vi "Begin.vi"(8 "error in":errorcluster) -> (0 "error out":errorcluster)   [LabVIEW 2016]
doc: "Called before other user functions, this VI is expected to open initial I/O refnums, load in file data, and do all program initialization. Notice that the <B>error out</B> terminal is simply used for data flow. Wiring it to other structures or subVIs ensures that this VI runs first."
uses:
  <vilib>/Rock Robotics/SystemInterfaces/i2clib/i2c_bus.ctl
  <vilib>/Rock Robotics/WPI/DriverStation/WPI_DriverStationRobotMode2.ctl
  <vilib>/Rock Robotics/WPI/Joystick/WPI_JoystickDeviceEnum.ctl
  <vilib>/Rock Robotics/SystemInterfaces/DIO/FPGA_DIOPWMChannel.ctl
  <vilib>/Rock Robotics/WPI/Solenoid/WPI_SolenoidChannel.ctl
  <vilib>/Rock Robotics/WPI/ThirdParty/CanMotor/TalonSRX/WPI_CANTalonSRX_APIControlMode.ctl
  Drive Commands.ctl
  FMS Commands.ctl
  Gear Command.ctl
  <vilib>/Rock Robotics/SystemInterfaces/DIO/FPGA_DIOChannel.ctl
  <userlib>/836-libraries/Drive/Drive_Code/Drive_Code_Support/Sensor_Cluster.ctl
  <userlib>/836-libraries/Drive/Drive_Code/Drive_Code_Support/Camera_Cluster.ctl
  <userlib>/836-libraries/Drive/Drive_Code/Drive_Code_Support/Drive_Code_Notifier.ctl
  <userlib>/836-libraries/Drive/Drive_Code/Drive_Code_Support/Drive_Code_Command.ctl
  <userlib>/836-libraries/Drive/Drive_Code/Logging_Data.ctl
  <userlib>/836-libraries/Drive/Drive_Code/Drive_Code_Support/Drive_Code_PID_Bundle.ctl
  <userlib>/836-libraries/Pneumatics/Support_Code/Pneumatics_Command.ctl
  <userlib>/836-libraries/Pneumatics/Support_Code/Pneumatics_Status.ctl
  <userlib>/836-libraries/Pneumatics/Support_Code/Pneumatics_Position.ctl
  <vilib>/Rock Robotics/WPI/Solenoid/WPI_SolenoidDevRef.ctl
  <vilib>/Rock Robotics/WPI/Solenoid/WPI_SolenoidValue.ctl
  Robot Global Data.vi
  <vilib>/Rock Robotics/WPI/RobotDrive/WPI_RobotDriveOpen4MotorWithVictorSP.vi
  <vilib>/Rock Robotics/WPI/MotorControl/WPI_MotorControlOpen Talon.vi
  <vilib>/Rock Robotics/WPI/Solenoid/WPI_SolenoidOpenDouble.vi
  <vilib>/Rock Robotics/WPI/Counter/WPI_CounterDigitalInputToDigitalSource.vi
  <vilib>/Rock Robotics/SystemInterfaces/AI/FPGA_AIChannel.ctl
  OpLightNotifier.ctl
panel:
  in  "I2C Bus Body IMU":T1=enum."I2C MXP"
  in  "I2C Bus Tur IMU":T1=enum."I2C MXP"
  in  "Calibrate?":bool
  out "Occupant Pri":u8[](array[numeric])=[160] format="%02x"
  out "Odd Pri":bool
  out "Odd Alt":bool
  out "Occupant Alt":u8[](array[numeric])=[160] format="%02x"
  in  "Gear Recv Init Pos":bool
  in  "Gear Shift Init Pos":bool=TRUE
  out "M 2":T2={"Boolean"=FALSE, "Boolean 2"=FALSE, "Boolean 3"=FALSE, "Boolean 4"=TRUE}
  out "A 2":T2={"Boolean"=TRUE, "Boolean 2"=FALSE, "Boolean 3"=FALSE, "Boolean 4"=FALSE}
  out "G 2":T2={"Boolean"=TRUE, "Boolean 2"=FALSE, "Boolean 3"=FALSE, "Boolean 4"=FALSE}
  out "S 2":T2={"Boolean"=FALSE, "Boolean 2"=FALSE, "Boolean 3"=FALSE, "Boolean 4"=TRUE}
  out "S":T2={"Boolean"=FALSE, "Boolean 2"=FALSE, "Boolean 3"=FALSE, "Boolean 4"=TRUE}
  out "G":T2={"Boolean"=TRUE, "Boolean 2"=FALSE, "Boolean 3"=FALSE, "Boolean 4"=FALSE}
  out "A":T2={"Boolean"=TRUE, "Boolean 2"=FALSE, "Boolean 3"=FALSE, "Boolean 4"=FALSE}
  out "M":T2={"Boolean"=FALSE, "Boolean 2"=FALSE, "Boolean 3"=FALSE, "Boolean 4"=TRUE}
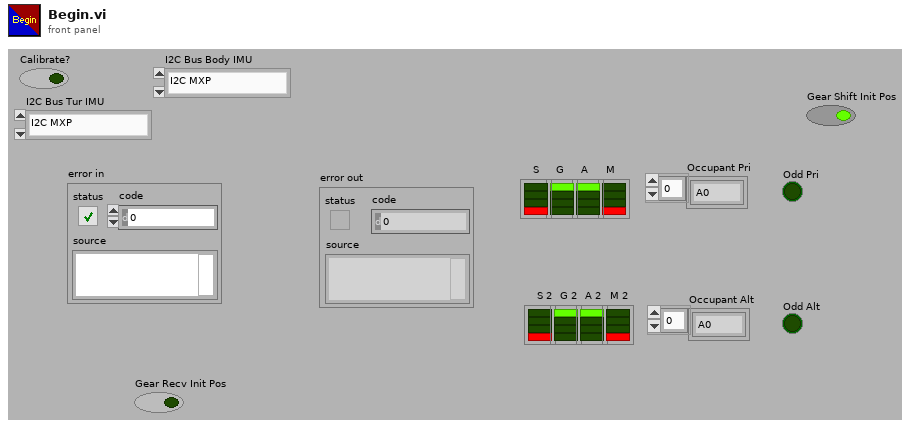
[diagram p1: front panel]
types:
  T1 = typedef "i2c_bus.ctl" = enum16{"I2C On-Board", "I2C MXP", "Invalid"}
  T2 = cluster{"Boolean":bool, "Boolean 2":bool, "Boolean 3":bool, "Boolean 4":bool}
  T3 = enum8{"ConfigMode", "AccOnly", "MagOnly", "GyroOnly", "AccMag", "AccGyro", "MagGyro", "AMG", "IMU", "Compass", "M4G", "NDOF_FMC_OFF", "NDOF"}
  T4 = typedef "FPGA_DIOPWMChannel.ctl" = enum8{"PWM 0", "PWM 1", "PWM 2", "PWM 3", "PWM 4", "PWM 5", "PWM 6", "PWM 7", "PWM 8", "PWM 9", "PWM MXP 0", "PWM MXP 1", "PWM MXP 2", "PWM MXP 3", "PWM MXP 4", "PWM MXP 5", "PWM MXP 6", "PWM MXP 7", "PWM MXP 8", "PWM MXP 9", "Invalid"}
  T5 = typedef "Gear Command.ctl" = enum16{"Home", "Floor Intake", "Catch", "Score"}
  T6 = typedef "WPI_JoystickDeviceEnum.ctl" = enum16{"USB 0", "USB 1", "USB 2", "USB 3", "USB 4", "USB 5"}
  T7 = typedef "FMS Commands.ctl" = enum16{"Shoot", "Un-Jam", "Stop"}
  T8 = typedef "Drive Commands.ctl" = enum16{"Manual", "Get Gear", "Score Gear", "Align Rope", "Turn To Angle", "Start Gear Score", "Place Gear", "Tank Drive", "Drive Distance"}
  T9 = typedef "WPI_CANTalonSRX_APIControlMode.ctl" = enum8{"Percent VBus", "Speed", "Position", "Slave", "Unchanged / Invalid", "Voltage Compensation", "Current", "Motion Profile", "Motion Magic"}
  T10 = typedef "WPI_SolenoidChannel.ctl" = enum8{"Solenoid 0", "Solenoid 1", "Solenoid 2", "Solenoid 3", "Solenoid 4", "Solenoid 5", "Solenoid 6", "Solenoid 7", "Invalid"}
  T11 = typedef "WPI_DriverStationRobotMode2.ctl" = enum16{"Autonomous Disabled", "Autonomous Enabled", "Teleop Disabled", "Teleop Enabled", "Disconnected", "Finish", "Test Disabled", "Test Enabled", "Emergency Stopped"}
  T12 = typedef "FPGA_AIChannel.ctl" = enum8{"AI 0", "AI 1", "AI 2", "AI 3", "AI MXP 0", "AI MXP 1", "AI MXP 2", "AI MXP 3", "Invalid"}
  T13 = typedef "FPGA_DIOChannel.ctl" = enum8{"DIO 0", "DIO 1", "DIO 2", "DIO 3", "DIO 4", "DIO 5", "DIO 6", "DIO 7", "DIO 8", "DIO 9", "DIO MXP 0", "DIO MXP 1", "DIO MXP 2", "DIO MXP 3", "DIO MXP 4", "DIO MXP 5", "DIO MXP 6", "DIO MXP 7", "DIO MXP 8", "DIO MXP 9", "DIO MXP 10", "DIO MXP 11", "DIO MXP 12", "DIO MXP 13", "DIO MXP 14", "DIO MXP 15", "SPI Port CS1", "SPI Port CS2", "SPI Port CS3", "SPI Port MISO", "SPI Port MOSI", "Invalid"}
  T14 = typedef "OpLightNotifier.ctl" = enum16{"Gears", " Balls", "Both"}
  T15 = typedef "WPI_I2CDevRef.ctl" = cluster{"DevStatus":errorcluster, "Device Address":u8, "Handle":i32, "I2C Bus":T1}
  T16 = cluster{"Cluster":cluster{"[0]":bool, "[1]":bool, "[2]":bool, "[3]":bool}, "Cluster":cluster{"[0]":bool, "[1]":bool, "[2]":bool, "[3]":bool}, "Cluster":cluster{"[0]":bool, "[1]":bool, "[2]":bool, "[3]":bool}, "Cluster":cluster{"[0]":bool, "[1]":bool, "[2]":bool, "[3]":bool}}
  T17 = cluster{"[0]":bool, "[1]":bool, "[2]":bool, "[3]":bool}
  T18 = typedef "WPI_JoystickDevRef.ctl" = cluster{"Device":T6}
  T19 = typedef "WPI_MotorControlDeviceRef.ctl" = cluster{"DeviceStatus":errorcluster, "Type":T20, "PWM":cluster{"PWM Channel":T4, "DeadBand":T21}, "CAN":cluster{"Device Number":u8, "SetOutput VI Ref":variant, "GetOutput VI Ref":variant, "Enable VI Ref":variant, "Disable VI Ref":variant, "Data":variant}, "Invert":bool}
  T20 = typedef "WPI_MotorControlType.ctl" = enum16{"PWM", "CAN"}
  T21 = typedef "WPI_PWMDeadband.ctl" = cluster{"Name":string, "maxPositivePwm":i32, "minPositivePwm":i32, "centerPwm":i32, "maxNegativePwm":i32, "minNegativePwm":i32, "angularRange":u16}
  T22 = typedef "WPI_RobotDriveDevRef.ctl" = cluster{"DevStatus":errorcluster, "Motors[]":T19[], "Square Inputs":bool, "Max Output":dbl}
  T23 = typedef "Drive_Code_Bundle.ctl" = cluster{"Sensor Data":T24, "Drive Command rt fifo":refnum<k33>, "Logging Data":refnum<k33>, "PID Update":refnum<notifier>}
  T24 = typedef "Sensor_Cluster.ctl" = cluster{"Gyro Data":cluster{"Gyro RT FIFO":refnum<k33>, "Gyro Current":dbl, "Gyro Hold":dbl}, "Encoder Data":cluster{"Encoder RT FIFO":refnum<k33>, "Encoder Current":dbl, "Encoder Hold":dbl}, "Camera Data":cluster{"Camera RT FIFO":refnum<k33>, "Camera Current":T25}}
  T25 = typedef "Camera_Cluster.ctl" = cluster{" Angle":dbl, "Valid":bool}
  T26 = typedef "WPI_SolenoidDevRef.ctl" = cluster{"DevStatus":errorcluster, "Pneumatics Control Module":u8, "Forward Solenoid Channel":T10, "Reverse Solenoid Channel":T10}
  T27 = typedef "Solenoid_Control_Loop.ctl" = cluster{"Control Notifier":refnum<notifier>, "Initial Position":T28, "SolenoidDevRef":T26, "Status Loop":refnum<k33>}
  T28 = typedef "Pneumatics_Position.ctl" = enum16{"Forward", "Reverse"}
  T29 = typedef "Pneumatics_Notifier.ctl" = cluster{"Command":refnum<notifier>, "Status":refnum<queue>}
  T30 = typedef "WPI_DigitalInputDevRef.ctl" = cluster{"DevStatus":errorcluster, "DIO Channel":T13}
  T31 = typedef "FPGA_CounterEncoderSourceConvertionLVSourceType.ctl" = cluster{"DevStatus":errorcluster, "AnalogTriggerMode?":bool, "DigitalMode":cluster{"DIO Channel":T32}, "AnalogTriggerMode":cluster{"AnalogTriggerIndex":T33, "OutputType":T34}}
  T32 = typedef "FPGA_DIODigitalSourceChannel.ctl" = enum8{"DIO 0", "DIO 1", "DIO 2", "DIO 3", "DIO 4", "DIO 5", "DIO 6", "DIO 7", "DIO 8", "DIO 9", "DIO MXP 0", "DIO MXP 1", "DIO MXP 2", "DIO MXP 3", "DIO MXP 4", "DIO MXP 5", "DIO MXP 6", "DIO MXP 7", "DIO MXP 8", "DIO MXP 9", "DIO MXP 10", "DIO MXP 11", "DIO MXP 12", "DIO MXP 13", "DIO MXP 14", "DIO MXP 15", "Disabled"}
  T33 = typedef "FPGA_AnalogTriggerIndex.ctl" = enum8{"Trig 0", "Trig 1", "Trig 2", "Trig 3", "Trig 4", "Trig 5", "Trig 6", "Trig 7", "Invalid"}
  T34 = typedef "FPGA_AnalogTriggerOutType.ctl" = enum16{"InWindow", "TriggerState", "Rising", "Falling"}
  T35 = typedef "WPI_EncoderDevRef.ctl" = cluster{"DevStatus":errorcluster, "EncoderIndex":T36, "CounterIndex":T37, "DistancePerCount":dbl, "Decoding Type":T38}
  T36 = typedef "FPGA_EncoderIdx.ctl" = enum8{"Enc 0", "Enc 1", "Enc 2", "Enc 3", "Enc 4", "Enc 5", "Enc 6", "Enc 7", "Invalid"}
  T37 = typedef "FPGA_CounterCtrSystemIndex.ctl" = enum8{"Ctr 0", "Ctr 1", "Ctr 2", "Ctr 3", "Ctr 4", "Ctr 5", "Ctr 6", "Ctr 7", "Invalid"}
  T38 = typedef "WPI_EncoderType.ctl" = enum16{"1x", "2x", "4x"}
  T39 = typedef "WPI_AnalogChannelDevRef.ctl" = cluster{"DevStatus":errorcluster, "Analog Channel":T12}
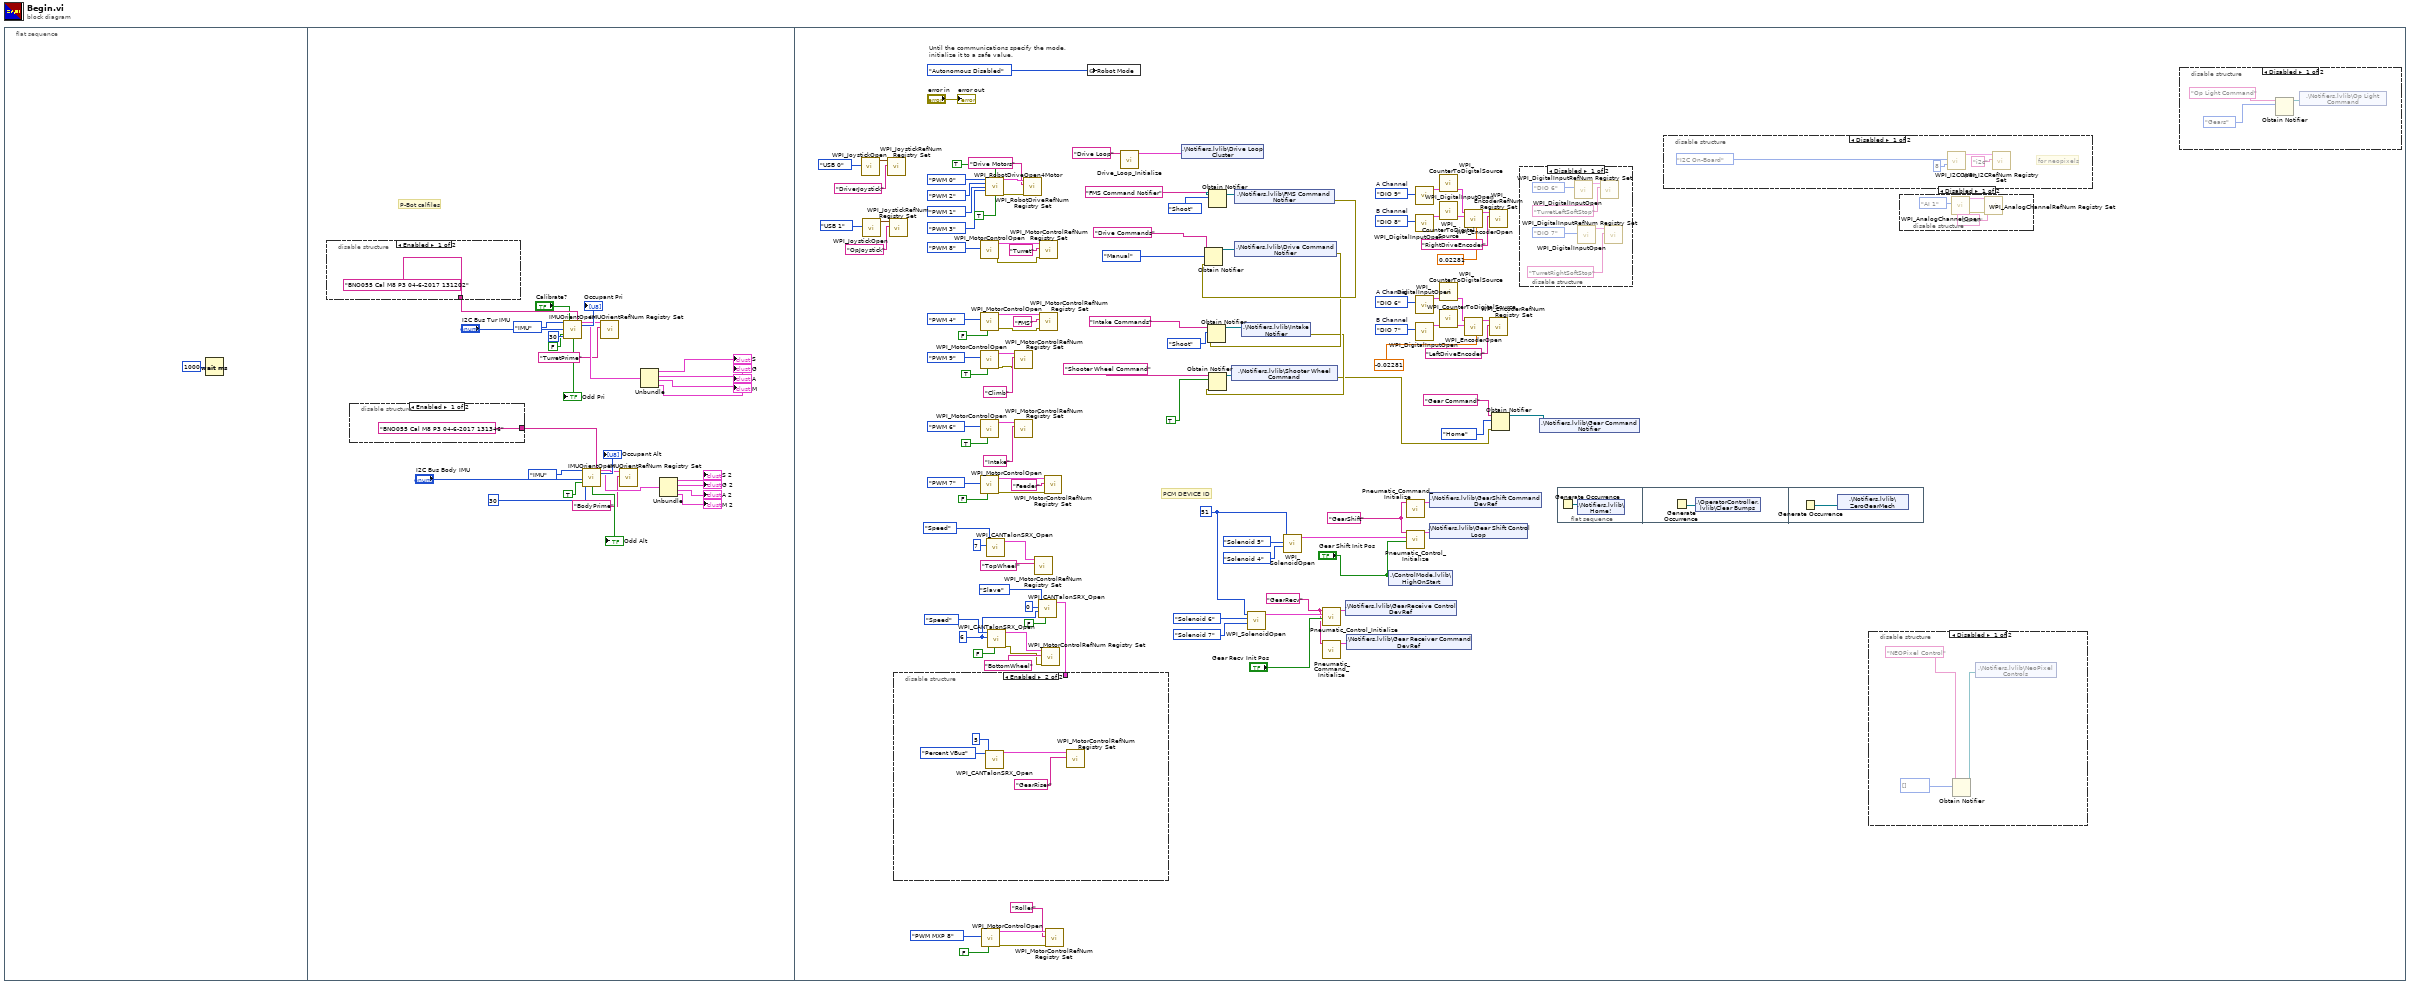
[diagram p0: block diagram]
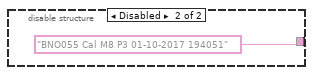
[diagram p2: hidden frame]
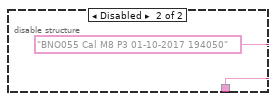
[diagram p3: hidden frame]
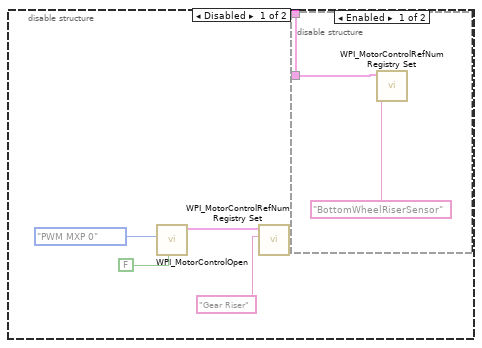
[diagram p7: hidden frame]
diagram:
  n1 = flat-sequence {
    frame #0 {
      n2 = Wait (ms)(milliseconds to wait=u32 1000) -> ()  [unwired: 1 out]
    }
    frame #1 {
      # "P-Bot calfiles"
      n3 = disable-structure shown="Enabled" {
        disable-tunnel: ["BNO055 Cal M8 P3 04-6-2017 131202" ("Stored Cal File") "BNO055 Cal M8 P3 01-10-2017 194050" ("Stored Cal File")] -> w29
        frame Enabled {
        }
        frame Disabled {
        }
      }
      n4 = disable-structure shown="Enabled" {
        disable-tunnel: ["BNO055 Cal M8 P3 04-6-2017 131346" ("Stored Cal File") "BNO055 Cal M8 P3 01-10-2017 194051" ("Stored Cal File")] -> w9
        frame Enabled {
        }
        frame Disabled {
        }
      }
      n5 = call <userlib>:"IMUOrientOpen.vi"("Op Mode"=T3."IMU", "Calibrate?"="Calibrate?", "Stored Cal File"=w29, "I2C Bus"="I2C Bus Tur IMU", "Status delay"=30, "Alt Adr?"=FALSE) -> ("Occupant"=→"Occupant Pri":u8[], "I2CDevRef"=w18:T15, "Cal Status @ Open"=w20:T16, "Odd"=→"Odd Pri":bool)  [unwired: 4 in, 2 out]
      n6 = call <userlib>:"IMUOrientOpen.vi"("Op Mode"=T3."IMU", "Stored Cal File"=w9, "I2C Bus"="I2C Bus Body IMU", "Status delay"=30, "Alt Adr?"=TRUE) -> ("Occupant"=→"Occupant Alt":u8[], "I2CDevRef"=w8:T15, "Cal Status @ Open"=w12:T16, "Odd"=→"Odd Alt":bool)  [unwired: 5 in, 2 out]
      n7 = call <userlib>:"IMUOrientRefNum Registry Set.vi"("refnum name"="TurretPrime", "I2CDevRef in"=w18) -> ()  [unwired: 8 in, 2 out]
      n8 = call <userlib>:"IMUOrientRefNum Registry Set.vi"("refnum name"="BodyPrime", "I2CDevRef in"=w8) -> ()  [unwired: 8 in, 2 out]
      n9 = Unbundle(w20) -> ("Cluster"=→"S":T17, "Cluster"=→"G":T17, "Cluster"=→"A":T17, "Cluster"=→"M":T17)
      n10 = Unbundle(w12) -> ("Cluster"=→"S 2":T17, "Cluster"=→"G 2":T17, "Cluster"=→"A 2":T17, "Cluster"=→"M 2":T17)
    }
    frame #2 {
      w49 = FPGA_DIOChannel."DIO 7"  # B Channel
      w48 = FPGA_DIOChannel."DIO 6"  # A Channel
      w57 = FPGA_DIOChannel."DIO 8"  # B Channel
      w56 = FPGA_DIOChannel."DIO 9"  # A Channel
      w89 = "GearRecv" ("Gearshift Control")
      w91 = "GearShift" ("Gearshift Control")
      w106 = u8 51 ("Pneumatics Control Module (0)")
      w114 = u8 6 ("Device Number")
      # "PCM DEVICE ID"
      # "Until the communications specify the mode,\ninitialize it to a safe value."
      n11 = call <vilib>:"WPI_JoystickOpen.vi"("JoystickDevice"=WPI_JoystickDeviceEnum."USB 0") -> ("JoystickDevRef"=w145:T18)  [unwired: 10 in]
      n12 = call <vilib>:"WPI_JoystickOpen.vi"("JoystickDevice"=WPI_JoystickDeviceEnum."USB 1") -> ("JoystickDevRef"=w75:T18)  [unwired: 10 in]
      n13 = call <vilib>:"WPI_JoystickRefNum Registry Set.vi"("refnum name"="DriverJoystick", "JoystickDevRef"=w145) -> ()  [unwired: 8 in, 2 out]
      n14 = call <vilib>:"WPI_JoystickRefNum Registry Set.vi"("refnum name"="OpJoystick", "JoystickDevRef"=w75) -> ()  [unwired: 8 in, 2 out]
      n15 = call-poly <vilib>:"WPI_MotorControlOpen.vi"("Invert"=FALSE, "PWM Channel"=FPGA_DIOPWMChannel."PWM 4") -> ("error out"=w62:errorcluster, "MotorControlDeviceRef"=w126:T19)  [unwired: 8 in]
      n16 = call-poly <vilib>:"WPI_MotorControlOpen.vi"("Invert"=TRUE, "PWM Channel"=FPGA_DIOPWMChannel."PWM 9") -> ("error out"=w60:errorcluster, "MotorControlDeviceRef"=w122:T19)  [unwired: 8 in]
      n17 = call-poly <vilib>:"WPI_MotorControlOpen.vi"("Invert"=TRUE, "PWM Channel"=FPGA_DIOPWMChannel."PWM 6") -> ("MotorControlDeviceRef"=w74:T19)  [unwired: 8 in, 1 out]
      n18 = call-poly <vilib>:"WPI_MotorControlOpen.vi"("Invert"=FALSE, "PWM Channel"=FPGA_DIOPWMChannel."PWM 7") -> ("error out"=w59:errorcluster, "MotorControlDeviceRef"=w124:T19)  [unwired: 8 in]
      n19 = call-poly <vilib>:"WPI_MotorControlOpen.vi"("PWM Channel"=FPGA_DIOPWMChannel."PWM 8") -> ("error out"=w63:errorcluster, "MotorControlDeviceRef"=w131:T19)  [unwired: 9 in]
      n20 = call-poly <vilib>:"WPI_MotorControlOpen.vi"("Invert"=FALSE, "PWM Channel"=FPGA_DIOPWMChannel."PWM MXP 8") -> ("error out"=w35:errorcluster, "MotorControlDeviceRef"=w39:T19)  [unwired: 8 in]
      n21 = call-poly <vilib>:"WPI_RobotDriveOpen4Motor.vi"("Rear Left Motor"=FPGA_DIOPWMChannel."PWM 0", "Rear Right Motor Inverted"=TRUE, "Rear Right Motor"=FPGA_DIOPWMChannel."PWM 2", "Front Left Motor"=FPGA_DIOPWMChannel."PWM 1", "Front Right Motor"=FPGA_DIOPWMChannel."PWM 3", "Front Right Motor Inverted"=TRUE) -> ("RobotDriveDevRef"=w138:T22, "error out"=w136:errorcluster)  [unwired: 8 in]
      n22 = call <vilib>:"WPI_CANTalonSRX_Open.vi"("Device Number"=u8 7, "Control Mode"=WPI_CANTalonSRX_APIControlMode."Speed") -> ("CAN Talon SRX Ref"=w108:T19)  [unwired: 8 in, 1 out]
      n23 = call <vilib>:"WPI_CANTalonSRX_Open.vi"("Invert"=FALSE, "Device Number"=w114, "Control Mode"=WPI_CANTalonSRX_APIControlMode."Speed") -> ("error out"=w61:errorcluster, "CAN Talon SRX Ref"=w117:T19)  [unwired: 7 in]
      n24 = call <vilib>:"WPI_MotorControlRefNum Registry Set.vi"("error in (no error)"=w60, "refnum name"="Climb", "MotorControlDevRef"=w122) -> ()  [unwired: 7 in, 2 out]
      n25 = call <vilib>:"WPI_MotorControlRefNum Registry Set.vi"("refnum name"="Intake", "MotorControlDevRef"=w74) -> ()  [unwired: 8 in, 2 out]
      n26 = call <vilib>:"WPI_RobotDriveRefNum Registry Set.vi"("error in (no error)"=w136, "refnum name"="Drive Motors", "RobotDriveDevRef"=w138) -> ()  [unwired: 7 in, 2 out]
      n27 = call <vilib>:"WPI_MotorControlRefNum Registry Set.vi"("refnum name"="TopWheel", "MotorControlDevRef"=w108) -> ()  [unwired: 8 in, 2 out]
      n28 = call <vilib>:"WPI_CANTalonSRX_Open.vi"("Invert"=FALSE, "Master Device Number"=w114, "Device Number"=u8 0, "Control Mode"=WPI_CANTalonSRX_APIControlMode."Slave") -> ("CAN Talon SRX Ref"=w70:T19)  [unwired: 6 in, 1 out]
      n29 = disable-structure shown="Enabled" {
        disable-tunnel: w70 -> [w162 _]
        frame Disabled {
          n30 = call-poly <vilib>:"WPI_MotorControlOpen.vi"("Invert"=FALSE, "PWM Channel"=FPGA_DIOPWMChannel."PWM MXP 0") -> ("MotorControlDeviceRef"=w163:T19)  [unwired: 8 in, 1 out]
          n31 = call <vilib>:"WPI_MotorControlRefNum Registry Set.vi"("refnum name"="Gear Riser", "MotorControlDevRef"=w163) -> ()  [unwired: 8 in, 2 out]
          n32 = disable-structure shown="Enabled" {
            disable-tunnel: w162 -> [w167 _]
            frame Enabled {
              n33 = call <vilib>:"WPI_MotorControlRefNum Registry Set.vi"("refnum name"="BottomWheelRiserSensor", "MotorControlDevRef"=w167) -> ()  [unwired: 8 in, 2 out]
            }
            frame Disabled {
            }
          }
        }
        frame Enabled {
          n34 = call <vilib>:"WPI_CANTalonSRX_Open.vi"("Device Number"=u8 5, "Control Mode"=WPI_CANTalonSRX_APIControlMode."Percent VBus") -> ("CAN Talon SRX Ref"=w170:T19)  [unwired: 8 in, 1 out]
          n35 = call <vilib>:"WPI_MotorControlRefNum Registry Set.vi"("refnum name"="GearRiser", "MotorControlDevRef"=w170) -> ()  [unwired: 8 in, 2 out]
        }
      }
      n36 = call <vilib>:"WPI_MotorControlRefNum Registry Set.vi"("error in (no error)"=w62, "refnum name"="FMS", "MotorControlDevRef"=w126) -> ()  [unwired: 7 in, 2 out]
      n37 = call <vilib>:"WPI_MotorControlRefNum Registry Set.vi"("error in (no error)"=w63, "refnum name"="Turret", "MotorControlDevRef"=w131) -> ()  [unwired: 7 in, 2 out]
      n38 = call <vilib>:"WPI_MotorControlRefNum Registry Set.vi"("error in (no error)"=w61, "refnum name"="BottomWheel", "MotorControlDevRef"=w117) -> ()  [unwired: 7 in, 2 out]
      n39 = call <vilib>:"WPI_MotorControlRefNum Registry Set.vi"("error in (no error)"=w59, "refnum name"="Feeder", "MotorControlDevRef"=w124) -> ()  [unwired: 7 in, 2 out]
      n40 = call <vilib>:"WPI_MotorControlRefNum Registry Set.vi"("error in (no error)"=w35, "refnum name"="Roller", "MotorControlDevRef"=w39) -> ()  [unwired: 7 in, 2 out]
      n41 = global write "Robot Global Data.vi" "Robot Mode"(WPI_DriverStationRobotMode2."Autonomous Disabled" ("Robot Mode")) -> ()
      n42 = call <userlib>:"Drive_Loop_Initialize.vi"("Name of drive loop (give it a name!)"="Drive Loop") -> ("Drive Loop Cluster"=w104:T23)  [unwired: 9 in, 1 out]
      n43 = shared-variable ".\\Notifiers.lvlib\\Drive Loop Cluster"(w104) -> ()  [unwired: 1 in, 1 out]
      n44 = Obtain Notifier(name (unnamed)="FMS Command Notifier", notification data type=FMS_Commands."Shoot") -> (notifier out=w93:refnum<notifier>)  [unwired: 2 in, 2 out]
      n45 = shared-variable ".\\Notifiers.lvlib\\FMS Command Notifier"(w93) -> (error out=w66:errorcluster)  [unwired: 1 in]
      n46 = Obtain Notifier(name (unnamed)="Drive Commands", notification data type=Drive_Commands."Manual", error in (no error)=w66) -> (notifier out=w103:refnum<notifier>)  [unwired: 1 in, 2 out]
      n47 = shared-variable ".\\Notifiers.lvlib\\Drive Command Notifier"(w103) -> (error out=w65:errorcluster)  [unwired: 1 in]
      n48 = Obtain Notifier(name (unnamed)="Intake Commands", notification data type=FMS_Commands."Shoot", error in (no error)=w65) -> (notifier out=w87:refnum<notifier>)  [unwired: 1 in, 2 out]
      n49 = shared-variable ".\\Notifiers.lvlib\\Intake Notifier"(w87) -> (error out=w64:errorcluster)  [unwired: 1 in]
      n50 = Obtain Notifier(name (unnamed)="Shooter Wheel Command", notification data type=TRUE, error in (no error)=w64) -> (notifier out=w78:refnum<notifier>)  [unwired: 1 in, 2 out]
      n51 = shared-variable ".\\Notifiers.lvlib\\Shooter Wheel Command"(w78) -> (error out=w58:errorcluster)  [unwired: 1 in]
      n52 = call-poly <vilib>:"WPI_SolenoidOpen.vi"("Reverse Solenoid Channel"=WPI_SolenoidChannel."Solenoid 7", "Forward Solenoid Channel"=WPI_SolenoidChannel."Solenoid 6", "Pneumatics Control Module (0)"=w106) -> ("SolenoidDevRef"=w95:T26)  [unwired: 7 in, 1 out]
      n53 = call-poly <vilib>:"WPI_SolenoidOpen.vi"("Reverse Solenoid Channel"=WPI_SolenoidChannel."Solenoid 4", "Forward Solenoid Channel"=WPI_SolenoidChannel."Solenoid 5" ("Solenoid Channel"), "Pneumatics Control Module (0)"=w106) -> ("SolenoidDevRef"=w99:T26)  [unwired: 7 in, 1 out]
      n54 = call <userlib>:"Pneumatic_Control_Initialize.vi"("Forward?"="Gear Recv Init Pos", "SolenoidDevRef"=w95, "name (unnamed)"=w89) -> ("Control Loop"=w94:T27)  [unwired: 7 in, 1 out]
      n55 = call <userlib>:"Pneumatic_Command_Initialize.vi"("name (unnamed)"=w89) -> ("Pneumatic Command Cluster"=w88:T29)  [unwired: 9 in, 1 out]
      n56 = shared-variable ".\\Notifiers.lvlib\\GearReceive Control DevRef"(w94) -> ()  [unwired: 1 in, 1 out]
      n57 = shared-variable ".\\Notifiers.lvlib\\Gear Receiver Command DevRef"(w88) -> ()  [unwired: 1 in, 1 out]
      n58 = shared-variable ".\\ControlMode.lvlib\\HighOnStart"("Gear Shift Init Pos") -> ()  [unwired: 1 in, 1 out]
      n59 = call <userlib>:"Pneumatic_Command_Initialize.vi"("name (unnamed)"=w91) -> ("Pneumatic Command Cluster"=w90:T29)  [unwired: 9 in, 1 out]
      n60 = call <userlib>:"Pneumatic_Control_Initialize.vi"("Forward?"="Gear Shift Init Pos", "SolenoidDevRef"=w99, "name (unnamed)"=w91) -> ("Control Loop"=w83:T27)  [unwired: 7 in, 1 out]
      n61 = call <vilib>:"WPI_DigitalInputOpen.vi"("DIO Channel"=w56) -> ("DigitalInputDevRef"=w53:T30)  [unwired: 1 in, 9 out]
      n62 = call <vilib>:"WPI_DigitalInputOpen.vi"("DIO Channel"=w57) -> ("DigitalInputDevRef"=w54:T30)  [unwired: 1 in, 9 out]
      n63 = call <vilib>:"WPI_DigitalInputOpen.vi"("DIO Channel"=w48) -> ("DigitalInputDevRef"=w45:T30)  [unwired: 1 in, 9 out]
      n64 = call <vilib>:"WPI_DigitalInputOpen.vi"("DIO Channel"=w49) -> ("DigitalInputDevRef"=w46:T30)  [unwired: 1 in, 9 out]
      n65 = shared-variable ".\\Notifiers.lvlib\\GearShift Command DevRef"(w90) -> ()  [unwired: 1 in, 1 out]
      n66 = shared-variable ".\\Notifiers.lvlib\\Gear Shift Control Loop"(w83) -> ()  [unwired: 1 in, 1 out]
      n67 = call-poly <vilib>:"WPI_CounterToDigitalSource.vi"("DigitalInputDevRef"=w53) -> ("Digital Source"=w52:T31)  [unwired: 6 out]
      n68 = call-poly <vilib>:"WPI_CounterToDigitalSource.vi"("DigitalInputDevRef"=w54) -> ("Digital Source"=w55:T31)  [unwired: 6 out]
      n69 = call-poly <vilib>:"WPI_CounterToDigitalSource.vi"("DigitalInputDevRef"=w45) -> ("Digital Source"=w44:T31)  [unwired: 6 out]
      n70 = call-poly <vilib>:"WPI_CounterToDigitalSource.vi"("DigitalInputDevRef"=w46) -> ("Digital Source"=w47:T31)  [unwired: 6 out]
      n71 = call <vilib>:"WPI_EncoderOpen.vi"("DistancePerCount"=0.02281, "BSource"=w55, "ASource"=w52) -> ("EncoderDevRef"=w51:T35)  [unwired: 5 in, 3 out]
      n72 = call <vilib>:"WPI_EncoderOpen.vi"("DistancePerCount"=-0.02281, "BSource"=w47, "ASource"=w44) -> ("EncoderDevRef"=w43:T35)  [unwired: 5 in, 3 out]
      n73 = call <vilib>:"WPI_EncoderRefNum Registry Set.vi"("refnum name"="RightDriveEncoder", "EncoderDevRef"=w51) -> ()  [unwired: 8 in, 2 out]
      n74 = call <vilib>:"WPI_EncoderRefNum Registry Set.vi"("refnum name"="LeftDriveEncoder", "EncoderDevRef"=w43) -> ()  [unwired: 8 in, 2 out]
      n75 = Obtain Notifier(name (unnamed)="Gear Command", notification data type=Gear_Command."Home", error in (no error)=w58) -> (notifier out=w67:refnum<notifier>)  [unwired: 1 in, 2 out]
      n76 = disable-structure shown="Disabled" {
        frame Disabled {
          n77 = call <vilib>:"WPI_DigitalInputOpen.vi"("DIO Channel"=FPGA_DIOChannel."DIO 6") -> ("DigitalInputDevRef"=w177:T30)  [unwired: 9 in, 1 out]
          n78 = call <vilib>:"WPI_DigitalInputOpen.vi"("DIO Channel"=FPGA_DIOChannel."DIO 7") -> ("DigitalInputDevRef"=w175:T30)  [unwired: 9 in, 1 out]
          n79 = call <vilib>:"WPI_DigitalInputRefNum Registry Set.vi"("refnum name"="TurretLeftSoftStop", "DigitalInputDevRef"=w177) -> ()  [unwired: 8 in, 2 out]
          n80 = call <vilib>:"WPI_DigitalInputRefNum Registry Set.vi"("refnum name"="TurretRightSoftStop", "DigitalInputDevRef"=w175) -> ()  [unwired: 8 in, 2 out]
        }
        frame Enabled {
        }
      }
      n81 = shared-variable ".\\Notifiers.lvlib\\Gear Command Notifier"(w67) -> ()  [unwired: 1 in, 1 out]
      n82 = flat-sequence {
        frame #0 {
          n83 = Generate Occurrence() -> (w156:refnum<k4>)
          n84 = shared-variable ".\\Notifiers.lvlib\\Home!"(w156) -> ()  [unwired: 1 in, 1 out]
        }
        frame #1 {
          n85 = Generate Occurrence() -> (w157:refnum<k4>)
          n86 = shared-variable ".\\OperatorController.lvlib\\Clear Bumps"(w157) -> ()  [unwired: 1 in, 1 out]
        }
        frame #2 {
          n87 = Generate Occurrence() -> (w158:refnum<k4>)
          n88 = shared-variable ".\\Notifiers.lvlib\\ZeroGearMech"(w158) -> ()  [unwired: 1 in, 1 out]
        }
      }
      n89 = disable-structure shown="Disabled" {
        frame Disabled {
          # "for neopixels"
          n90 = call <vilib>:"WPI_I2COpen.vi"("Device Address"=u8 8, "I2C Bus"=i2c_bus."I2C On-Board") -> ("I2CDevRef"=w155:T15)  [unwired: 8 in, 1 out]
          n91 = call <vilib>:"WPI_I2CRefNum Registry Set.vi"("refnum name"="i2c", "I2CDevRef"=w155) -> ()  [unwired: 8 in, 2 out]
        }
        frame Enabled {
        }
      }
      n92 = disable-structure shown="Disabled" {
        frame Disabled {
          n93 = Obtain Notifier(name (unnamed)="NEOPixel Control", notification data type=u8[] []) -> (notifier out=w159:refnum<notifier>)  [unwired: 2 in, 2 out]
          n94 = shared-variable ".\\Notifiers.lvlib\\NeoPixel Controls"(w159) -> ()  [unwired: 1 in, 1 out]
        }
        frame Enabled {
        }
      }
      n95 = disable-structure shown="Disabled" {
        frame Disabled {
          n96 = call <vilib>:"WPI_AnalogChannelOpen.vi"("Analog Channel"=FPGA_AIChannel."AI 1") -> ("error out"=w150:errorcluster, "AIDeviceRef"=w149:T39)  [unwired: 9 in]
          n97 = call <vilib>:"WPI_AnalogChannelRefNum Registry Set.vi"("error in (no error)"=w150, "refnum name"="Sonar", "AIDeviceRef"=w149) -> ()  [unwired: 7 in, 2 out]
        }
        frame Enabled {
        }
      }
      n98 = disable-structure shown="Disabled" {
        frame Disabled {
          n99 = Obtain Notifier(name (unnamed)="Op Light Command", notification data type=OpLightNotifier."Gears") -> (notifier out=w179:refnum<notifier>)  [unwired: 2 in, 2 out]
          n100 = shared-variable ".\\Notifiers.lvlib\\Op Light Command"(w179) -> ()  [unwired: 1 in, 1 out]
        }
        frame Enabled {
        }
      }
      "error out" <- "error in"
    }
  }
